vi "conexion_buk_vi.vi"() -> ()   [LabVIEW 2014]
uses:
  <vilib>/Instr/_visa.llb/VISA Open Access Mode.ctl
  <vilib>/Instr/_visa.llb/VISA Configure Serial Port (Instr).vi
panel:
  in  "Slide":u8(slide) scale=0.0..255.0
  out "before substring":string
  in  "Stop Button":bool
  in  "VISA resource name":refnum<visa-resource-name>
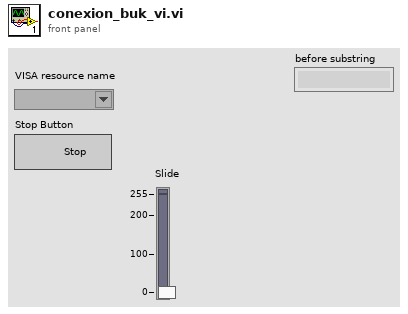
[diagram p1: front panel]
types:
  T1 = typedef "VISA Open Access Mode.ctl" = u32
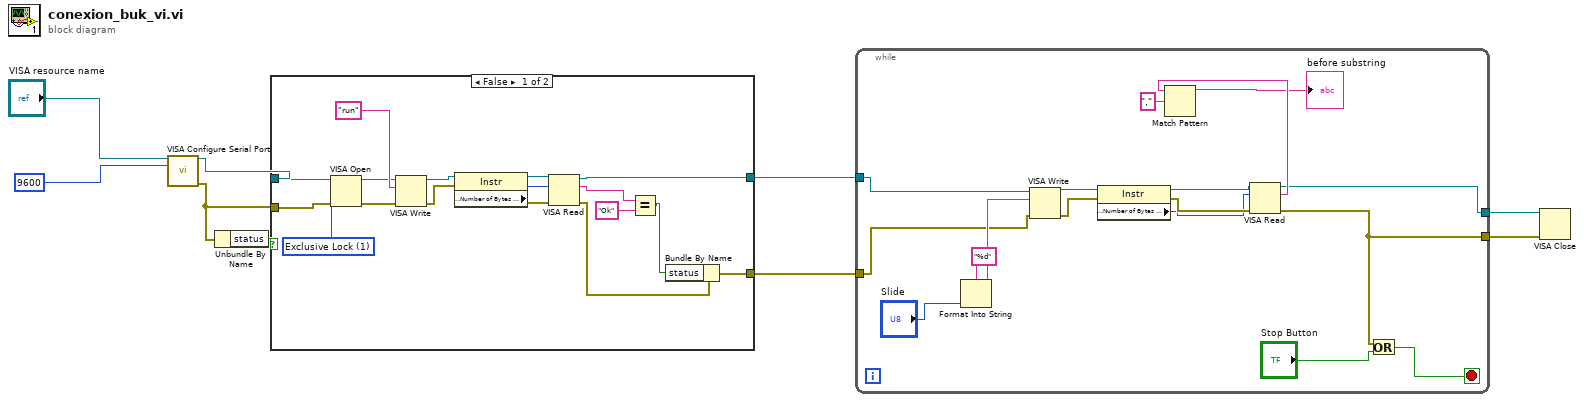
[diagram p0: block diagram]
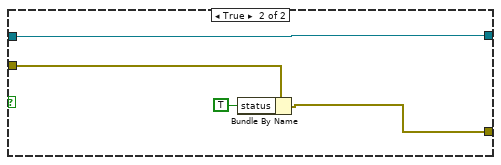
[diagram p2: hidden frame]
diagram:
  n1 = call-poly "VISA Configure Serial Port"("VISA resource name"="VISA resource name", "baud rate (9600)"=u32 9600) -> ("VISA resource name out"=w7:refnum<visa-resource-name>, "error out"=w8:errorcluster)  [unwired: 12 in]
  n2 = Unbundle By Name(w8) -> ("status"=w9:bool)
  n3 = case shown="False" w9 {
    tunnel: w8 -> [w22 w30]
    tunnel: w7 -> [w23 w28]
    tunnel: [w21 w28] -> w3
    tunnel: [w17 w27] -> w4
    frame False {
      w10 = T1 1 items=["VISA Defaults"=0, "Exclusive Lock"=1, "Load Configured Settings"=4] ("Access Mode")
      n4 = VISA Open(access mode=w10, error in (no error)=w22, VISA resource name=w23) -> (VISA resource name=w12:refnum<visa-resource-name>, error out=w11:errorcluster)  [unwired: 2 in]
      n5 = VISA Write(VISA resource name=w12, write buffer="run", error in (no error)=w11) -> (VISA resource name out=w15:refnum<visa-resource-name>, error out=w14:errorcluster)  [unwired: 1 out]
      n6 = property class="Instr"(reference=w15, error in=w14) -> (reference out=w24:refnum<visa-resource-name>, error out=w26:errorcluster, "Serial Settings:Number of Bytes at Serial Port"=w25:u32)
      n7 = VISA Read(VISA resource name=w24, byte count=w25, error in (no error)=w26) -> (VISA resource name out=w21:refnum<visa-resource-name>, read buffer=w20:string, error out=w18:errorcluster)  [unwired: 1 out]
      n8 = Equal?(x=w20, y="Ok") -> (x = y?=w16:bool)
      n9 = Bundle By Name(cluster=w18, "status"=w16) -> (w17:errorcluster)
    }
    frame True {
      n10 = Bundle By Name(cluster=w30, "status"=TRUE) -> (w27:errorcluster)
    }
  }
  n11 = while {
    tunnel: w4 -> [w36]
    tunnel: w3 -> [w35]
    tunnel: [w32] -> w1
    tunnel: [w31] -> w2
    stop <- w47 stop-if-true
    n12 = Format Into String(format string="%d", "Slide") -> (resulting string=w38:string)  [unwired: 2 in, 1 out]
    n13 = VISA Write(VISA resource name=w35, write buffer=w38, error in (no error)=w36) -> (VISA resource name out=w33:refnum<visa-resource-name>, error out=w34:errorcluster)  [unwired: 1 out]
    n14 = property class="Instr"(reference=w33, error in=w34) -> (reference out=w45:refnum<visa-resource-name>, error out=w44:errorcluster, "Serial Settings:Number of Bytes at Serial Port"=w43:u32)
    n15 = VISA Read(VISA resource name=w45, byte count=w43, error in (no error)=w44) -> (VISA resource name out=w31:refnum<visa-resource-name>, read buffer=w42:string, error out=w32:errorcluster)  [unwired: 1 out]
    n16 = Match Pattern(string=w42, regular expression=",") -> (before substring=→"before substring":string)  [unwired: 1 in, 3 out]
    n17 = Or(x=w32, y="Stop Button") -> (x .or. y?=w47:bool)
  }
  n18 = VISA Close(VISA resource name=w2, error in (no error)=w1) -> ()  [unwired: 1 out]
